vi "New Stat Section with Sort.vi"(0 "Stats In":string[][](array[string]), 7 "DataPt In":string[](array[string]), 11 "CMDCluster In":T1) -> (4 "Stats Out":string[][](array[string]), 15 "PrevDataIndex":i32)   [LabVIEW 2013]
uses:
  TypeDef/Command Cluster.ctl
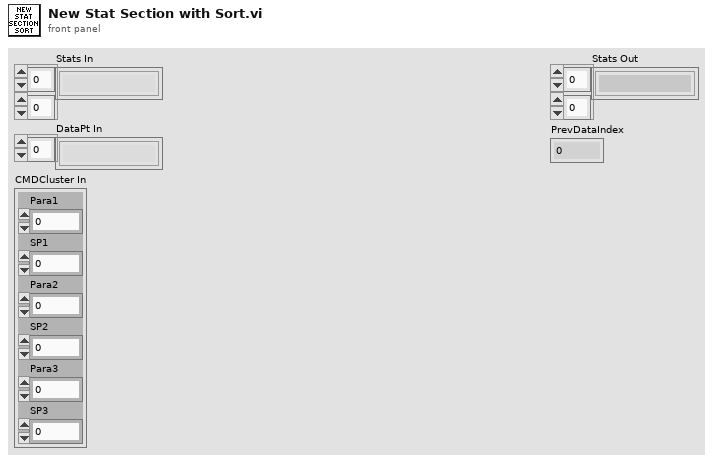
[diagram p1: front panel]
types:
  T1 = typedef "Command Cluster.ctl" = cluster{"Para1":i32, "SP1":dbl, "Para2":i32, "SP2":dbl, "Para3":i32, "SP3":dbl}
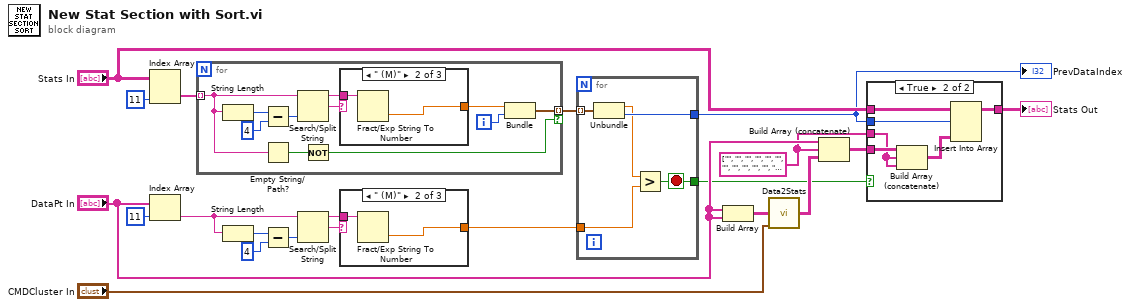
[diagram p0: block diagram]
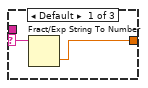
[diagram p2: hidden frame]
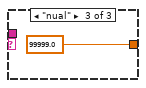
[diagram p3: hidden frame]
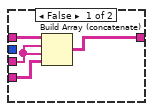
[diagram p4: hidden frame]
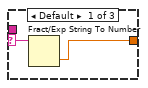
[diagram p5: hidden frame]
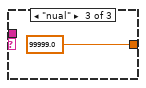
[diagram p6: hidden frame]
diagram:
  w8 = string[] ["", "", "", "", "", "", "", "", "", "", "", "", "", ""]
  n1 = Index Array(array="Stats In", index (col)=11 ("disabled index (col)")) -> (element=w19:string[])  [unwired: 1 in]
  n2 = Index Array(array="DataPt In", index=11) -> (element=w2:string)
  n3 = for {
    tunnel: w19 -> [w27] mode=indexing
    tunnel: [w24] -> w18 mode=indexing if=w22
    i -> [w25]
    n4 = String Length(string=w27) -> (length=w32:i32)
    n5 = Subtract(x=w32, y=4) -> (x-y=w29:i32)
    n6 = Empty String/Path?(string/path=w27) -> (empty?=w23:bool)
    n7 = Search/Split String(string=w27, offset (0)=w29) -> (substring before match=w28:string, match + rest of string=w30:string)  [unwired: 1 in, 1 out]
    n8 = Not(x=w23) -> (.not. x?=w22:bool)
    n9 = case shown="\" (M)\"" w30 {
      selector: w30 -> [w34 _ _]
      tunnel: [w33 w35 99999.0] -> w26
      tunnel: w28 -> [_ w36 _]
      frame Default {
        n10 = Fract/Exp String To Number(string=w34) -> (number=w33:dbl)  [unwired: 3 in, 1 out]
      }
      frame " (M)" {
        n11 = Fract/Exp String To Number(string=w36) -> (number=w35:dbl)  [unwired: 3 in, 1 out]
      }
      frame "nual" {
      }
    }
    n12 = Bundle(w26, w25) -> (w24:cluster{dbl, i32})  [unwired: 1 in]
  }
  n13 = String Length(string=w2) -> (length=w3:i32)
  n14 = Subtract(x=w3, y=4) -> (x-y=w6:i32)
  n15 = Search/Split String(string=w2, offset (0)=w6) -> (substring before match=w7:string, match + rest of string=w5:string)  [unwired: 1 in, 1 out]
  n16 = case shown="\" (M)\"" w5 {
    selector: w5 -> [w39 _ _]
    tunnel: [w38 w40 99999.0] -> w1
    tunnel: w7 -> [_ w41 _]
    frame Default {
      n17 = Fract/Exp String To Number(string=w39) -> (number=w38:dbl)  [unwired: 3 in, 1 out]
    }
    frame " (M)" {
      n18 = Fract/Exp String To Number(string=w41) -> (number=w40:dbl)  [unwired: 3 in, 1 out]
    }
    frame "nual" {
    }
  }
  n19 = for {
    tunnel: w18 -> [w47] mode=indexing
    tunnel: w1 -> [w44]
    tunnel: [w46] -> w11
    tunnel: [w43] -> w9
    stop <- w43 stop-if-true
    n20 = Unbundle(w47) -> (w45:dbl, w46:i32)
    n21 = Greater?(x=w45, y=w44) -> (0:w43:bool)
  }
  "PrevDataIndex" <- w11
  n22 = Build Array("DataPt In", "DataPt In") -> (w17:string[][])
  n23 = call "Data2Stats.vi"("DataIn"=w17, "DesiredParameters"="CMDCluster In") -> ("StatsOut"=w16:string[][])  [unwired: 13 in]
  n24 = Build Array (concatenate)("DataPt In", w8, w16) -> (w13:string[][])
  n25 = case shown="True" w9 {
    tunnel: "Stats In" -> [w51 w57]
    tunnel: w13 -> [w49 w54]
    tunnel: [w50 w56] -> w12
    tunnel: w11 -> [_ w55]
    tunnel: w8 -> [w48 w53]
    frame False {
      n26 = Build Array (concatenate)(w51, w48, w48, w49) -> (w50:string[][])
    }
    frame True {
      n27 = Build Array (concatenate)(w54, w53, w53) -> (w52:string[][])
      n28 = Insert Into Array(array=w57, index (row)=w55, new element=w52) -> (w56:string[][])  [unwired: 1 in]
    }
  }
  "Stats Out" <- w12
